vi "WebServiceData_Init.vi"(0 "reference in":refnum<class "WebServiceData.lvclass"> caption="This control should only be used when\na sub class is inheriting this class", 5 "error in (no error)":errorcluster) -> (14 "reference out":refnum<class "WebServiceData.lvclass"> caption="This indicator should only be used when\na sub class is inheriting this class", 19 "error out":errorcluster)   [LabVIEW 2019, in "WebServiceData.lvclass"]
uses:
  WebServiceData.lvclass
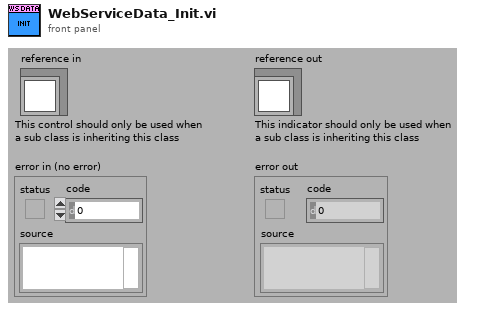
[diagram p1: front panel]
types:
  T1 = typedef "WebServiceData.lvclass/ObjectAttributes.ctl" = cluster{"ActualValues":cluster{"T":dbl, "RH":dbl}}
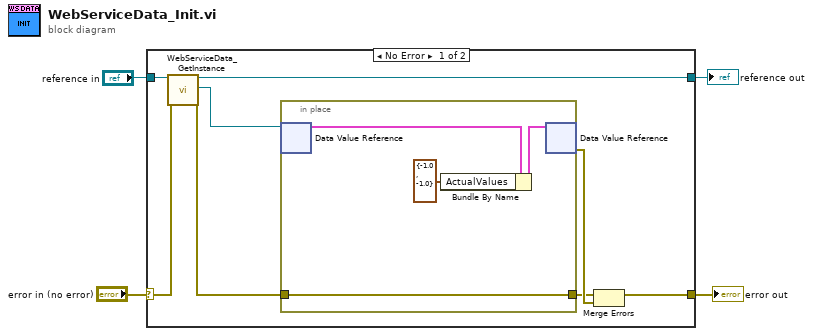
[diagram p0: block diagram]
diagram:
  n1 = case shown="No Error" "error in (no error)" {
    selector: "error in (no error)" -> [w10 w18]
    tunnel: [w11 w18] -> w3
    tunnel: "reference in" -> [w9 w17]
    tunnel: [w8 w17] -> w1
    frame No Error {
      n2 = call "WebServiceData_GetInstance.vi"("reference in"=w9, "error in (no error)"=w10) -> ("reference out"=w8:refnum<class "WebServiceData.lvclass">, "DVRRefOut"=w7:refnum<data-value>, "error out"=w6:errorcluster)  [unwired: 13 in, 2 out]
      n3 = in-place {
        in-place-border: w6 -> [w14]
        in-place-border: [w14] -> w5
        n4 = in-place-dvr #1(w7) -> (w15:T1)  [unwired: 1 out]
        n5 = Bundle By Name(cluster=w15, "ActualValues"=cluster{"T":dbl, "RH":dbl} {"T"=-1.0, "RH"=-1.0}) -> (w16:T1)
        n6 = in-place-dvr #1(w16) -> (w12:errorcluster)  [unwired: 1 out]
      }
      n7 = Merge Errors(w5, w12) -> (w11:errorcluster)
    }
    frame Error {
    }
  }
  "error out" <- w3
  "reference out" <- w1
